vi "testing_SRS_VI_parts.vi"() -> ()   [LabVIEW 2011]
panel:
  out "read buffer":string
  in  "output":u16(ring) items=["T0", "A", "B", "AB", "C", "D", "CD"]
  out "write string":string
  in  "VISA resource name":refnum<visa-resource-name>
  out "error out":errorcluster
  in  "stop":bool
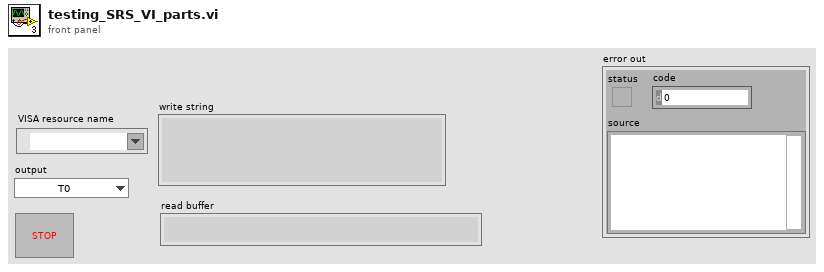
[diagram p1: front panel]
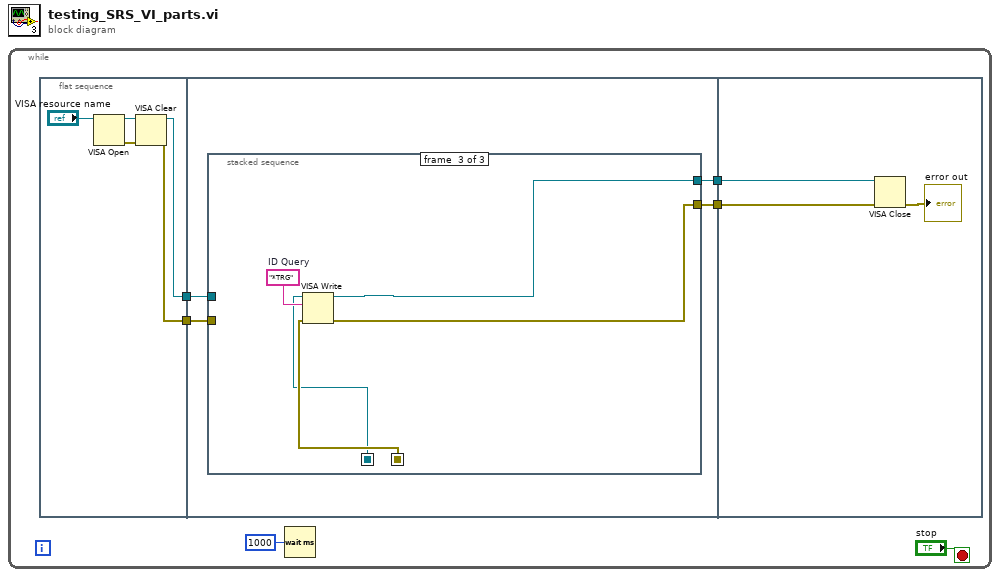
[diagram p0: block diagram]
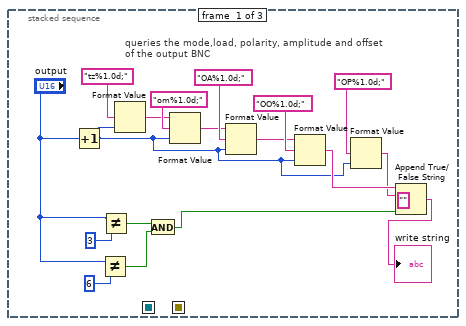
[diagram p2: hidden frame]
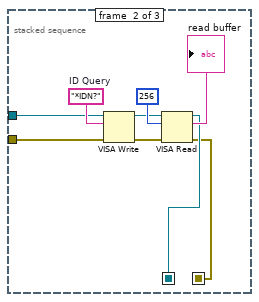
[diagram p3: hidden frame]
diagram:
  n1 = while {
    stop <- "stop" stop-if-true
    n2 = flat-sequence {
      tunnel: [w8] -> w5
      tunnel: [w7] -> w4
      tunnel: w5 -> [w15]
      tunnel: w4 -> [w14]
      tunnel: [w13] -> w2
      tunnel: [w12] -> w1
      tunnel: w2 -> [w50]
      tunnel: w1 -> [w49]
      frame #0 {
        n3 = VISA Open(VISA resource name="VISA resource name") -> (VISA resource name=w11:refnum<visa-resource-name>, error out=w10:errorcluster)  [unwired: 4 in]
        n4 = VISA Clear(VISA resource name=w11, error in (no error)=w10) -> (VISA resource name out=w8:refnum<visa-resource-name>, error out=w7:errorcluster)
      }
      frame #1 {
        n5 = stacked-sequence {
          seq-local: [_ w36 _] -> [_ _ w46]
          seq-local: [_ w35 _] -> [_ _ w47]
          tunnel: w15 -> [_ w38 _]
          tunnel: w14 -> [_ w37 _]
          tunnel: [_ _ w44] -> w13
          tunnel: [_ _ w45] -> w12
          frame #0 {
            # "queries the mode,load, polarity, amplitude and offset\nof the output BNC"
            n6 = Increment(x="output") -> (x+1=w18:u16)
            n7 = Not Equal?(x="output", y=6) -> (x != y?=w19:bool)
            n8 = Not Equal?(x="output", y=3) -> (x != y?=w27:bool)
            n9 = Format Value(format string="tz%1.0d;", value (0)=w18) -> (output string=w20:string)  [unwired: 1 in]
            n10 = And(x=w27, y=w19) -> (x .and. y?=w30:bool)
            n11 = Format Value(string ("")=w20, format string="om%1.0d;", value (0)=w18) -> (output string=w24:string)
            n12 = Format Value(string ("")=w24, format string="OA%1.0d;", value (0)=w18) -> (output string=w23:string)
            n13 = Format Value(string ("")=w23, format string="OO%1.0d;", value (0)=w18) -> (output string=w22:string)
            n14 = Format Value(format string="OP%1.0d;", value (0)=w18) -> (output string=w17:string)  [unwired: 1 in]
            n15 = Append True/False String(1:w30, 2:"", 3:w17, 4:w22) -> (0:→"write string":string)
          }
          frame #1 {
            w39 = "*IDN?"  # ID Query
            n16 = VISA Write(VISA resource name=w38, write buffer=w39, error in (no error)=w37) -> (VISA resource name out=w41:refnum<visa-resource-name>, error out=w40:errorcluster)  [unwired: 1 out]
            n17 = VISA Read(VISA resource name=w41, byte count=u32 256, error in (no error)=w40) -> (VISA resource name out=w36:refnum<visa-resource-name>, read buffer=→"read buffer":string, error out=w35:errorcluster)  [unwired: 1 out]
          }
          frame #2 {
            w48 = "*TRG"  # ID Query
            n18 = VISA Write(VISA resource name=w46, write buffer=w48, error in (no error)=w47) -> (VISA resource name out=w45:refnum<visa-resource-name>, error out=w44:errorcluster)  [unwired: 1 out]
          }
        }
      }
      frame #2 {
        n19 = VISA Close(VISA resource name=w49, error in (no error)=w50) -> (error out=→"error out":errorcluster)
      }
    }
    n20 = Wait (ms)(milliseconds to wait=u32 1000) -> ()  [unwired: 1 out]
  }
